vi "Autonomous.vi"   [LabVIEW 2019]
doc: "This VI starts when autonomous period begins, and will automatically be terminated when it ends. You can carry out timed or sensor driven operations directly to I/O or to subsystems without needing to return to the caller."
uses:
  <vilib>/Rock Robotics/WPI/Solenoid/WPI_SolenoidValue.ctl
  <vilib>/Rock Robotics/Network Tables/NT Read String.vi
  Framework/Robot Global Data.vi
types:
  T1 = typedef "WPI_SolenoidValue.ctl" = enum16{"Off", "On", "Forward", "Reverse"}
  T2 = typedef "Command Status Info.ctl" = cluster{"Name":string, "Status":T3, "notifier out":T4}
  T3 = typedef "Completion Status.ctl" = enum16{"Successful", "Aborted", "Incomplete"}
  T4 = typedef "Completion Notifier.ctl" = refnum<notifier>
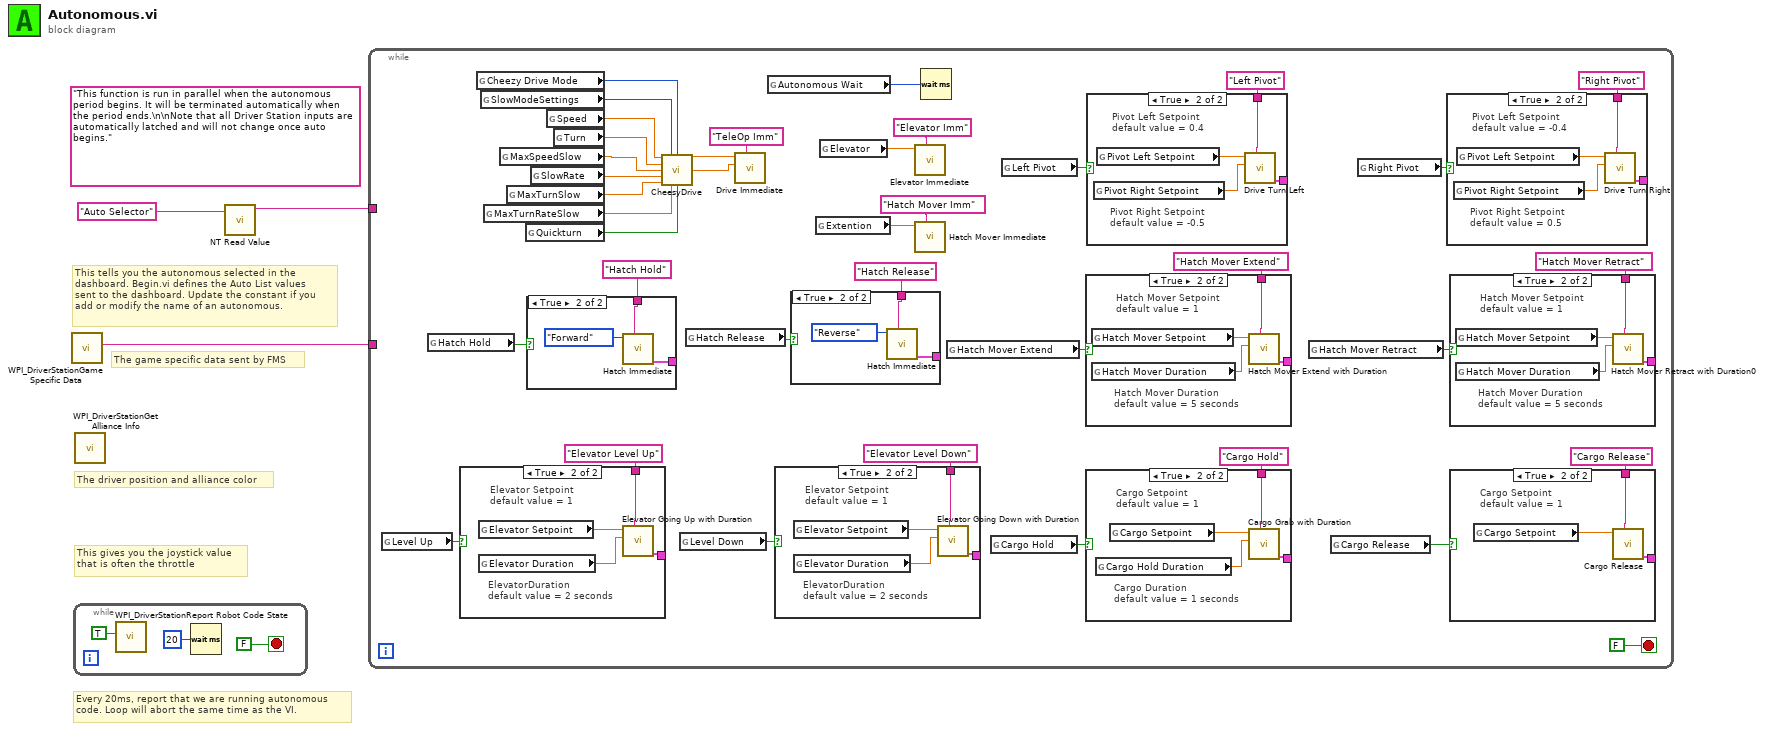
[diagram p0: block diagram]
diagram:
  (unwired) "This function is run in parallel when the autonomous period begins. It will be terminated automatically when the period ends.\n\nNote that all Driver Station inputs are automatically latched and will not change once auto begins."
  # "The game specific data sent by FMS"
  # "This tells you the autonomous selected in the \ndashboard. Begin.vi defines the Auto List values\nsent to the dashboard. Update the constant if you\nadd or modify the name of an autonomous."
  # "Every 20ms, report that we are running autonomous\ncode. Loop will abort the same time as the VI."
  # "This gives you the joystick value\nthat is often the throttle"
  # "The driver position and alliance color"
  n1 = call <vilib>:"WPI_DriverStationGame Specific Data.vi"() -> ("Game Specific Data"=w1:string)  [unwired: 11 in]
  n2 = while {
    stop <- FALSE stop-if-true
    n3 = call <vilib>:"WPI_DriverStationReport Robot Code State.vi"("Autonomous"=TRUE) -> ()  [unwired: 10 in, 1 out]
    n4 = Wait (ms)(milliseconds to wait=u32 20) -> ()  [unwired: 1 out]
  }
  n5 = call <vilib>:"WPI_DriverStationGet Alliance Info.vi"() -> ()  [unwired: 12 out]
  n6 = call-poly <vilib>:"NT Read Value.vi"("Name"="Auto Selector") -> ("String"=w2:string)  [unwired: 9 in, 1 out]
  n7 = while {
    tunnel: w2 -> [_]
    tunnel: w1 -> [_]
    stop <- FALSE stop-if-true
    n8 = global read "Robot Global Data.vi" "Level Up"() -> (w28:bool)
    n9 = global read "Robot Global Data.vi" "Hatch Hold"() -> (w13:bool)
    n10 = case shown="True" w28 {
      tunnel: "Elevator Level Up" ("Description") -> [_ w52]
      tunnel: [_ w49] -> _
      frame False {
      }
      frame True {
        # "ElevatorDuration\ndefault value = 2 seconds"
        # "Elevator Setpoint\ndefault value = 1"
        n11 = global read "Robot Global Data.vi" "Elevator Setpoint"() -> (w51:dbl)
        n12 = global read "Robot Global Data.vi" "Elevator Duration"() -> (w50:dbl)
        n13 = call "Elevator Going Up with Duration.vi"("Description"=w52, "Duration (s)"=w50, "Setpoint"=w51) -> ("Command Info Out"=w49:T2)  [unwired: 8 in]
      }
    }
    n14 = global read "Robot Global Data.vi" "Cheezy Drive Mode"() -> (w32:u32)
    n15 = global read "Robot Global Data.vi" "SlowModeSettings"() -> (w33:i32)
    n16 = global read "Robot Global Data.vi" "MaxTurnRateSlow"() -> (w39:dbl)
    n17 = global read "Robot Global Data.vi" "MaxSpeedSlow"() -> (w36:dbl)
    n18 = global read "Robot Global Data.vi" "MaxTurnSlow"() -> (w38:dbl)
    n19 = global read "Robot Global Data.vi" "Quickturn"() -> (w40:bool)
    n20 = case shown="True" w13 {
      tunnel: [_ w80] -> _
      tunnel: "Hatch Hold" ("Description") -> [_ w79]
      frame False {
      }
      frame True {
        n21 = call "Hatch Immediate.vi"("Description"=w79, "Action"=WPI_SolenoidValue."Forward") -> ("Command Info Out"=w80:T2)  [unwired: 9 in]
      }
    }
    n22 = global read "Robot Global Data.vi" "SlowRate"() -> (w37:dbl)
    n23 = global read "Robot Global Data.vi" "Speed"() -> (w34:dbl)
    n24 = global read "Robot Global Data.vi" "Turn"() -> (w35:dbl)
    n25 = call "CheesyDrive.vi"("Throttle"=w34, "SlowModeSettings"=w33, "SlowMode"=w32, "Wheel"=w35, "MaxSpeedSlow"=w36, "SlowRate"=w37, "MaxTurnSlow"=w38, "MaxTurnRateSlow"=w39, "Quickturn"=w40) -> ("Left PWM"=w41:dbl, "Right PWM"=w42:dbl)  [unwired: 5 in]
    n26 = global read "Robot Global Data.vi" "Level Down"() -> (w31:bool)
    n27 = global read "Robot Global Data.vi" "Hatch Release"() -> (w14:bool)
    n28 = call "Drive Immediate.vi"("Description"="TeleOp Imm", "Right Setpoint"=w42, "Left Setpoint"=w41) -> ()  [unwired: 8 in, 1 out]
    n29 = global read "Robot Global Data.vi" "Autonomous Wait"() -> (w9:u32)
    n30 = case shown="True" w31 {
      tunnel: "Elevator Level Down" ("Description") -> [_ w48]
      tunnel: [_ w45] -> _
      frame False {
      }
      frame True {
        # "ElevatorDuration\ndefault value = 2 seconds"
        # "Elevator Setpoint\ndefault value = 1"
        n31 = global read "Robot Global Data.vi" "Elevator Setpoint"() -> (w47:dbl)
        n32 = global read "Robot Global Data.vi" "Elevator Duration"() -> (w46:dbl)
        n33 = call "Elevator Going Down with Duration.vi"("Description"=w48, "Duration (s)"=w46, "Setpoint"=w47) -> ("Command Info Out"=w45:T2)  [unwired: 8 in]
      }
    }
    n34 = case shown="True" w14 {
      tunnel: [_ w77] -> _
      tunnel: "Hatch Release" ("Description") -> [_ w76]
      frame False {
      }
      frame True {
        n35 = call "Hatch Immediate.vi"("Description"=w76, "Action"=WPI_SolenoidValue."Reverse") -> ("Command Info Out"=w77:T2)  [unwired: 9 in]
      }
    }
    n36 = global read "Robot Global Data.vi" "Extention"() -> (w8:dbl)
    n37 = global read "Robot Global Data.vi" "Elevator"() -> (w44:dbl)
    n38 = call "Elevator Immediate.vi"("Description"="Elevator Imm", "Setpoint"=w44) -> ()  [unwired: 9 in, 1 out]
    n39 = call "Hatch Mover Immediate.vi"("Description"="Hatch Mover Imm", "Setpoint"=w8) -> ()  [unwired: 9 in, 1 out]
    n40 = Wait (ms)(milliseconds to wait=w9) -> ()  [unwired: 1 out]
    n41 = global read "Robot Global Data.vi" "Hatch Mover Extend"() -> (w20:bool)
    n42 = global read "Robot Global Data.vi" "Cargo Hold"() -> (w25:bool)
    n43 = global read "Robot Global Data.vi" "Left Pivot"() -> (w17:bool)
    n44 = case shown="True" w20 {
      tunnel: "Hatch Mover Extend" ("Description") -> [_ w67]
      tunnel: [_ w64] -> _
      frame False {
      }
      frame True {
        # "Hatch Mover Duration\ndefault value = 5 seconds"
        # "Hatch Mover Setpoint\ndefault value = 1"
        n45 = global read "Robot Global Data.vi" "Hatch Mover Setpoint"() -> (w66:dbl)
        n46 = global read "Robot Global Data.vi" "Hatch Mover Duration"() -> (w65:dbl)
        n47 = call "Hatch Mover Extend with Duration.vi"("Description"=w67, "Duration (s)"=w65, "Setpoint"=w66) -> ("Command Info Out"=w64:T2)  [unwired: 8 in]
      }
    }
    n48 = case shown="True" w25 {
      tunnel: "Cargo Hold" ("Description") -> [_ w59]
      tunnel: [_ w56] -> _
      frame False {
      }
      frame True {
        # "Cargo Duration\ndefault value = 1 seconds"
        # "Cargo Setpoint\ndefault value = 1"
        n49 = global read "Robot Global Data.vi" "Cargo Hold Duration"() -> (w57:dbl)
        n50 = global read "Robot Global Data.vi" "Cargo Setpoint"() -> (w58:dbl)
        n51 = call "Cargo Grab with Duration.vi"("Description"=w59, "Duration (s)"=w57, "Setpoint"=w58) -> ("Command Info Out"=w56:T2)  [unwired: 8 in]
      }
    }
    n52 = case shown="True" w17 {
      tunnel: "Left Pivot" ("Description") -> [_ w75]
      tunnel: [_ w72] -> _
      frame False {
      }
      frame True {
        # "Pivot Right Setpoint\ndefault value = -0.5"
        # "Pivot Left Setpoint\ndefault value = 0.4"
        n53 = global read "Robot Global Data.vi" "Pivot Right Setpoint"() -> (w73:dbl)
        n54 = global read "Robot Global Data.vi" "Pivot Left Setpoint"() -> (w74:dbl)
        n55 = call "Drive Turn Left.vi"("Description"=w75, "Right Setpoint"=w73, "Left Setpoint"=w74) -> ("Command Info Out"=w72:T2)  [unwired: 8 in]
      }
    }
    n56 = global read "Robot Global Data.vi" "Hatch Mover Retract"() -> (w23:bool)
    n57 = global read "Robot Global Data.vi" "Cargo Release"() -> (w26:bool)
    n58 = global read "Robot Global Data.vi" "Right Pivot"() -> (w18:bool)
    n59 = case shown="True" w18 {
      tunnel: "Right Pivot" ("Description") -> [_ w71]
      tunnel: [_ w68] -> _
      frame False {
      }
      frame True {
        # "Pivot Right Setpoint\ndefault value = 0.5"
        # "Pivot Left Setpoint\ndefault value = -0.4"
        n60 = global read "Robot Global Data.vi" "Pivot Right Setpoint"() -> (w69:dbl)
        n61 = global read "Robot Global Data.vi" "Pivot Left Setpoint"() -> (w70:dbl)
        n62 = call "Drive Turn Right.vi"("Description"=w71, "Right Setpoint"=w69, "Left Setpoint"=w70) -> ("Command Info Out"=w68:T2)  [unwired: 8 in]
      }
    }
    n63 = case shown="True" w23 {
      tunnel: "Hatch Mover Retract" ("Description") -> [_ w63]
      tunnel: [_ w60] -> _
      frame False {
      }
      frame True {
        # "Hatch Mover Duration\ndefault value = 5 seconds"
        # "Hatch Mover Setpoint\ndefault value = 1"
        n64 = global read "Robot Global Data.vi" "Hatch Mover Setpoint"() -> (w62:dbl)
        n65 = global read "Robot Global Data.vi" "Hatch Mover Duration"() -> (w61:dbl)
        n66 = call "Hatch Mover Retract with Duration0.vi"("Description"=w63, "Duration (s)"=w61, "Setpoint"=w62) -> ("Command Info Out"=w60:T2)  [unwired: 8 in]
      }
    }
    n67 = case shown="True" w26 {
      tunnel: "Cargo Release" ("Description") -> [_ w55]
      tunnel: [_ w53] -> _
      frame False {
      }
      frame True {
        # "Cargo Setpoint\ndefault value = 1"
        n68 = global read "Robot Global Data.vi" "Cargo Setpoint"() -> (w54:dbl)
        n69 = call "Cargo Release.vi"("Description"=w55, "Setpoint"=w54) -> ("Command Info Out"=w53:T2)  [unwired: 9 in]
      }
    }
  }
